vi "XML ( Clone and Append ).vi"   [LabVIEW 2018, in "XML.lvlib" / "XML.lvclass"]
uses:
  XML.lvclass
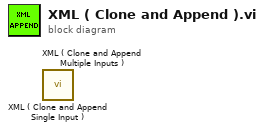
[diagram p0: block diagram]
diagram:
  n1 = call "XML ( Clone and Append Single Input ).vi"() -> ()  [unwired: 10 in, 2 out]
  n2 = call "XML ( Clone and Append Multiple Inputs ).vi"() -> ()  [unwired: 10 in, 2 out]
